vi "Measurement.Free.TestLauncher.vi"() -> ()   [LabVIEW 2017]
doc: "JKI State Machine Objects (SMO) 1.0.0.5\nJKI - JKI\nCopyright (c) 2016, JKI"
uses:
  Measurement.Free.UI.lvclass
  D:/Program Files (x86)/National Instruments/LabVIEW 2017/vi.lib/JKI/JKI SMO/SMO/SMO.lvclass
  D:/Program Files (x86)/National Instruments/LabVIEW 2017/vi.lib/JKI/JKI SMO/SMO.UI/SMO.UI.lvclass
  Measurement.Free/Measurement.Free.lvclass
  D:/upwork/Laser Measurement Tool/Laser/project/Subsystems/Measurement/Measurement.lvclass
  Measurement.Free/Typedefs/Configuration--Cluster.ctl
  Measurement.Free/Typedefs/Configuration.Hardware--Cluster.ctl
  Measurement/Typedefs/Configuration.SMU--Cluster.ctl
  SMU/Typedefs/Configuration--Cluster.ctl
  Measurement/Typedefs/Configuration.LIA--Cluster.ctl
  LIA/Typedefs/Configuration--Cluster.ctl
  Measurement/Typedefs/Configuration.OPM--Cluster.ctl
  OPM/Typedefs/Configuration--Cluster.ctl
  Measurement/Typedefs/Configuration.OPA--Cluster.ctl
  OPA/Typedefs/Configuration--Cluster.ctl
  <vilib>/JKI/JKI SMO/SMO/SMO.lvclass
  <vilib>/JKI/JKI SMO/SMO.UI/SMO.UI.lvclass
  OPA/OPA.lvclass
  Measurement/Measurement.lvclass
  OPM/OPM.lvclass
  LIA/LIA.lvclass
  SMU/SMU.lvclass
  <vilib>/Utility/config.llb/NI_LVConfig.lvlib
panel:
  in  "Configuration File Switch":bool=TRUE
  in  "Stop":bool
  # "Measurement.Free.TestLauncher"
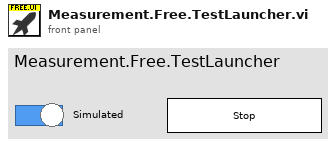
[diagram p1: front panel]
types:
  T1 = typedef "Measurement.Free.lvclass/Configuration--Cluster.ctl" = cluster{"Measurement.Type":enum16{"Free", "I/V Curve", "Wavelength sweeping", "Photocurrent mapping"}, "Hardware":T2}
  T2 = typedef "Measurement.Free.lvclass/Configuration.Hardware--Cluster.ctl" = cluster{"SMU":T3, "LIA":T5, "OPM":T7, "OPA":T9}
  T3 = typedef "Measurement.lvclass/Configuration.SMU--Cluster.ctl" = cluster{"Enable":bool, "SMU Model":string, "Configuration":T4}
  T4 = typedef "SMU.lvclass/Configuration--Cluster.ctl" = cluster{"VISA Resource":string, "Channel":string}
  T5 = typedef "Measurement.lvclass/Configuration.LIA--Cluster.ctl" = cluster{"Enable":bool, "LIA Model":string, "Configuration":T6}
  T6 = typedef "LIA.lvclass/Configuration--Cluster.ctl" = cluster{"VISA Resource":string}
  T7 = typedef "Measurement.lvclass/Configuration.OPM--Cluster.ctl" = cluster{"Enable":bool, "OPM Model":string, "Configuration":T8}
  T8 = typedef "OPM.lvclass/Configuration--Cluster.ctl" = cluster{"VISA Resource":string}
  T9 = typedef "Measurement.lvclass/Configuration.OPA--Cluster.ctl" = cluster{"Enable":bool, "OPA Model":string, "Configuration":T10}
  T10 = typedef "OPA.lvclass/Configuration--Cluster.ctl" = cluster{"Serial Number":string}
  T11 = typedef "NI_LVConfig.lvlib/Config Data RefNum.ctl" = refnum<k1>
  T12 = cluster{"SMO out":refnum<class "Measurement.Free.lvclass">}
  T13 = typedef "SMO.lvclass/Public Events.ctl" = cluster{"Error":refnum<user-event>, "State":refnum<user-event>, "Reserve State":refnum<user-event>}
  T14 = cluster{"SMO.UI Public Events":refnum<event-registration>, "Event Registration Refnum":refnum<event-registration>}
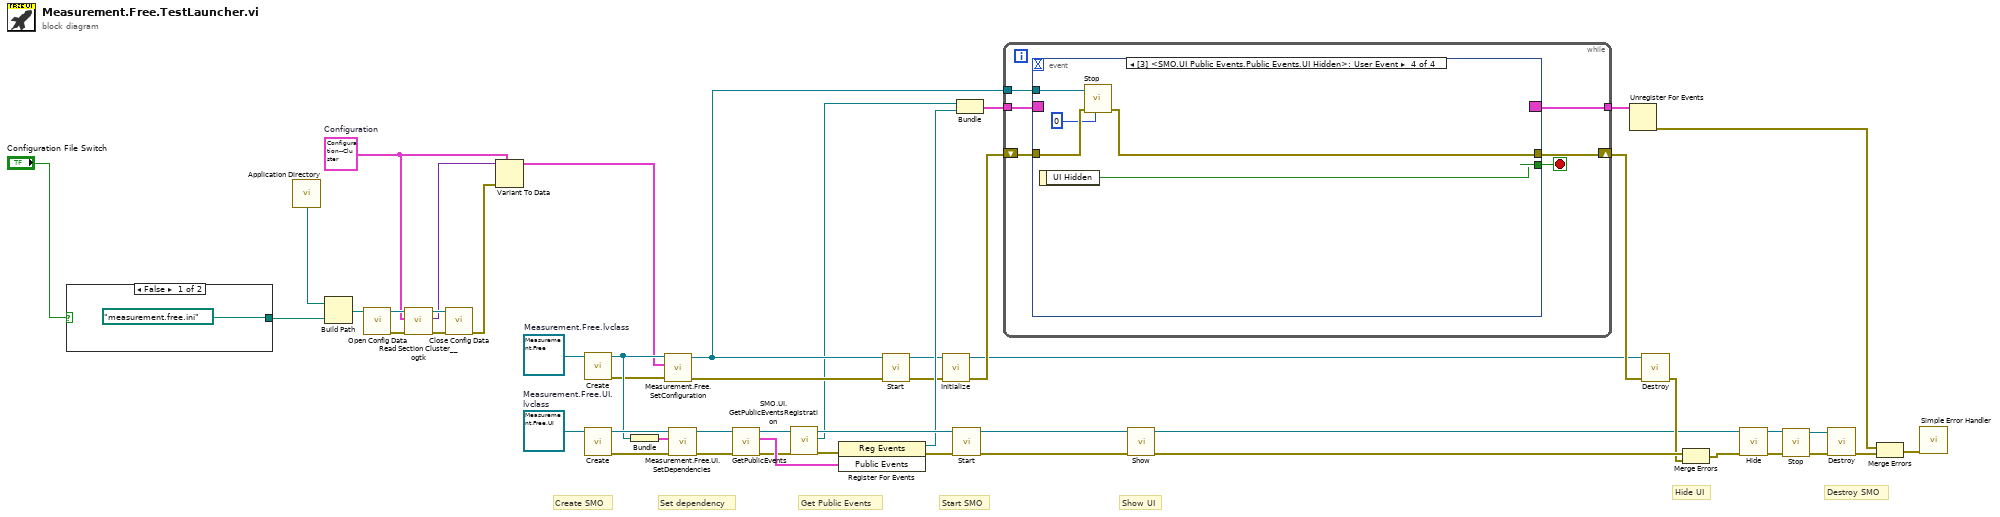
[diagram p0: block diagram]
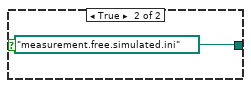
[diagram p2: hidden frame]
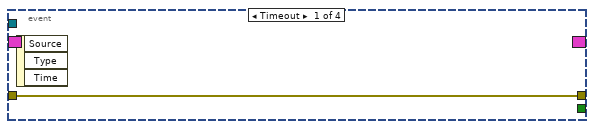
[diagram p3: hidden frame]
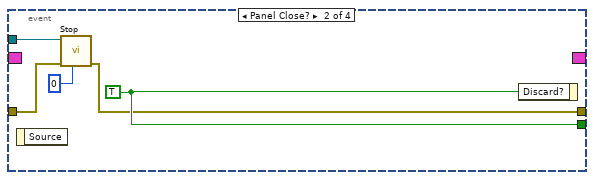
[diagram p4: hidden frame]
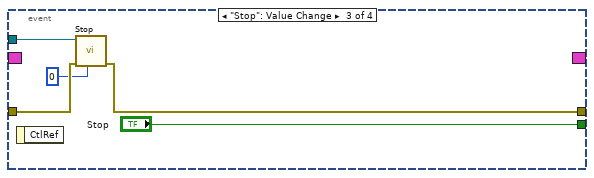
[diagram p5: hidden frame]
diagram:
  w7 = T1 {"Measurement.Type"=enum."Free", "Hardware"={"SMU"={"Enable"=FALSE, "SMU Model"="", "Configuration"={"VISA Resource"="", "Channel"=""}}, "LIA"={"Enable"=FALSE, "LIA Model"="", "Configuration"={"VISA Resource"=""}}, "OPM"={"Enable"=FALSE, "OPM Model"="", "Configuration"={"VISA Resource"=""}}, "OPA"={"Enable"=FALSE, "OPA Model"="", "Configuration"={"Serial Number"=""}}}}  # Configuration
  w43 = refnum<class "Measurement.Free.lvclass"> refnum  # Measurement.Free.lvclass
  w44 = refnum<class "Measurement.Free.UI.lvclass"> refnum  # Measurement.Free.UI.lvclass
  # "Set dependency"
  # "Hide UI"
  # "Show UI"
  # "Get Public Events"
  # "Start SMO"
  # "Destroy SMO"
  # "Create SMO"
  n1 = case shown="False" "Configuration File Switch" {
    tunnel: [path "measurement.free.ini" path "measurement.free.simulated.ini"] -> w15
    frame False {
    }
    frame True {
    }
  }
  n2 = call <vilib>:"Application Directory.vi"() -> ("Application Directory"=w16:path)
  n3 = Build Path(base path=w16, name or relative path=w15) -> (appended path=w14:path)
  n4 = call <vilib>:"Open Config Data.vi"("configuration file path"=w14) -> ("error out"=w13:errorcluster, "refnum"=w12:T11)  [unwired: 8 in, 1 out]
  n5 = call <userlib>:"Read Section Cluster__ogtk.vi"("error in (no error)"=w13, "Section Formatted Cluster Type"=w7, "refnum"=w12) -> ("error out"=w10:errorcluster, "Section Formatted Cluster"=w9:variant, "dup refnum"=w11:T11)  [unwired: 4 in, 2 out]
  n6 = call <vilib>:"Close Config Data.vi"("error in (no error)"=w10, "refnum"=w11) -> ("error out"=w8:errorcluster)  [unwired: 8 in, 1 out]
  n7 = Variant To Data(error in=w8, type=w7, Variant=w9) -> (data=w6:T1)  [unwired: 1 out]
  n8 = call <vilib>:"Create.vi"("SMO"=w43) -> ("error out"=w36:errorcluster, "SMO out"=w37:refnum<class "Measurement.Free.lvclass">)  [unwired: 8 in, 1 out]
  n9 = call <vilib>:"Create.vi"("SMO"=w44) -> ("error out"=w40:errorcluster, "SMO out"=w42:refnum<class "Measurement.Free.UI.lvclass">)  [unwired: 8 in, 1 out]
  n10 = Bundle("SMO out"=w37) -> (w41:T12)  [unwired: 1 in]
  n11 = call "Measurement.Free.SetConfiguration.vi"("error in (no error)"=w36, "Configuration"=w6, "Measurement.Free"=w37) -> ("error out"=w23:errorcluster, "Measurement.Free out"=w24:refnum<class "Measurement.Free.lvclass">)  [unwired: 7 in]
  n12 = call "Measurement.Free.UI.SetDependencies.vi"("error in (no error)"=w40, "Dependencies"=w41, "Measurement.Free.UI in"=w42) -> ("error out"=w38:errorcluster, "Measurement.Free.UI out"=w39:refnum<class "Measurement.Free.UI.lvclass">)  [unwired: 7 in]
  n13 = call <vilib>:"GetPublicEvents.vi"("error in (no error)"=w38, "SMO"=w39) -> ("error out"=w21:errorcluster, "Public Events"=w45:T13, "SMO out"=w22:refnum<class "Measurement.Free.UI.lvclass">)  [unwired: 7 in]
  n14 = call <vilib>:"SMO.UI.GetPublicEventsRegistration.vi"("error in (no error)"=w21, "SMO.UI"=w22) -> ("error out"=w19:errorcluster, "SMO.UI Public Events"=w17:refnum<event-registration>, "SMO.UI out"=w20:refnum<class "Measurement.Free.UI.lvclass">)  [unwired: 7 in]
  n15 = register-events(error in=w19, w45) -> (reference out=w18:refnum<event-registration>, error out=w46:errorcluster)  [unwired: 1 in]
  n16 = call <vilib>:"Start.vi"("error in (no error)"=w23, "SMO"=w24) -> ("error out"=w3:errorcluster, "SMO out"=w4:refnum<class "Measurement.Free.lvclass">)  [unwired: 8 in]
  n17 = call "Initialize.vi"("error in (no error)"=w3, "Measurement in"=w4) -> ("error out"=w2:errorcluster, "Measurement out"=w1:refnum<class "Measurement.Free.lvclass">)  [unwired: 8 in]
  n18 = call <vilib>:"Start.vi"("error in (no error)"=w46, "SMO"=w20) -> ("error out"=w48:errorcluster, "SMO out"=w49:refnum<class "Measurement.Free.UI.lvclass">)  [unwired: 8 in]
  n19 = Bundle("SMO.UI Public Events"=w17, "Event Registration Refnum"=w18) -> (w35:T14)  [unwired: 1 in]
  n20 = while {
    shift-right: [w58] -> w33
    shift-left: w2 -> [w57]
    tunnel: w35 -> [w54]
    tunnel: [w56] -> w34
    tunnel: w24 -> [w55]
    stop <- w59 stop-if-true
    n21 = event shown="[3] <SMO.UI Public Events.Public Events.UI Hidden>: User Event" {
      selector: w54 -> [_ _ _ _]
      dyn-events: [_ _ _ _] -> w56
      timeout: _ -> [_ _ _ _]
      tunnel: [_ w65 "Stop" w71] -> w59
      tunnel: w55 -> [_ w64 w69 w75]
      tunnel: [w60 w61 w67 w73] -> w58
      tunnel: w57 -> [w60 w62 w68 w74]
      event Timeout {
        n22 = event-data() -> ()  [unwired: 1 in, 3 out]
      }
      event Panel Close? {
        w65 = TRUE ("OK")
        n23 = event-data() -> ()  [unwired: 1 in, 1 out]
        n24 = call <vilib>:"Stop.vi"("timeout in ms (-1)"=0, "error in (no error)"=w62, "SMO"=w64) -> ("error out"=w61:errorcluster)  [unwired: 7 in, 1 out]
        n25 = event-data("Discard?"=w65) -> ()  [unwired: 1 in, 1 out]
      }
      event "Stop": Value Change {
        n26 = event-data() -> ()  [unwired: 1 in, 1 out]
        n27 = call <vilib>:"Stop.vi"("timeout in ms (-1)"=0, "error in (no error)"=w68, "SMO"=w69) -> ("error out"=w67:errorcluster)  [unwired: 7 in, 1 out]
      }
      event User Event {
        n28 = event-data() -> ("UI Hidden"=w71:bool)  [unwired: 1 in]
        n29 = call <vilib>:"Stop.vi"("timeout in ms (-1)"=0, "error in (no error)"=w74, "SMO"=w75) -> ("error out"=w73:errorcluster)  [unwired: 7 in, 1 out]
      }
    }
  }
  n30 = call <vilib>:"Show.vi"("error in (no error)"=w48, "SMO.UI"=w49) -> ("error out"=w47:errorcluster, "SMO.UI out"=w31:refnum<class "Measurement.Free.UI.lvclass">)  [unwired: 8 in]
  n31 = Unregister For Events(event registration refnum=w34) -> (error out=w51:errorcluster)  [unwired: 1 in]
  n32 = call <vilib>:"Destroy.vi"("error in (no error)"=w33, "SMO"=w1) -> ("error out"=w32:errorcluster)  [unwired: 9 in]
  n33 = Merge Errors(w47, w32) -> (w30:errorcluster)
  n34 = call <vilib>:"Hide.vi"("error in (no error)"=w30, "SMO.UI"=w31) -> ("error out"=w28:errorcluster, "SMO.UI out"=w29:refnum<class "Measurement.Free.UI.lvclass">)  [unwired: 8 in]
  n35 = call <vilib>:"Stop.vi"("error in (no error)"=w28, "SMO"=w29) -> ("error out"=w27:errorcluster, "SMO out"=w26:refnum<class "Measurement.Free.UI.lvclass">)  [unwired: 8 in]
  n36 = call <vilib>:"Destroy.vi"("error in (no error)"=w27, "SMO"=w26) -> ("error out"=w50:errorcluster)  [unwired: 9 in]
  n37 = Merge Errors(w51, w50) -> (w25:errorcluster)
  n38 = call <vilib>:"Simple Error Handler.vi"("error in (no error)"=w25) -> ()  [unwired: 4 in, 5 out]
